vi "Euler Check.vi"(8 "F(X,t)":string[](array[string]), 9 "X":string[](array[string]), 10 "time":string, 11 "X(0)":dbl[](array[numeric]) format="%.2f") -> (0 "system OK":bool, 1 "error text":string[](array[string]), 2 "error":i32[](array[numeric]), 3 "error message":string, 4 "result":dbl[][](array[numeric]), 5 "table":i32[][][](array[numeric]))   [LabVIEW 2014, in "NI_Gmath.lvlib"]
uses:
  NI_Gmath.lvlib
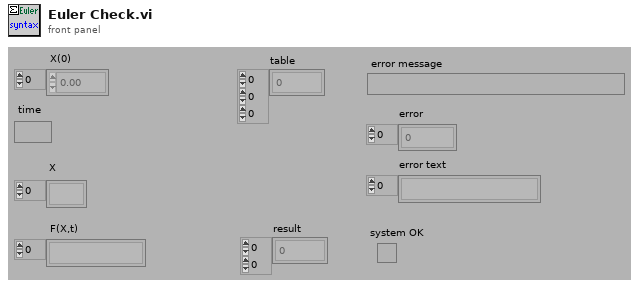
[diagram p1: front panel]
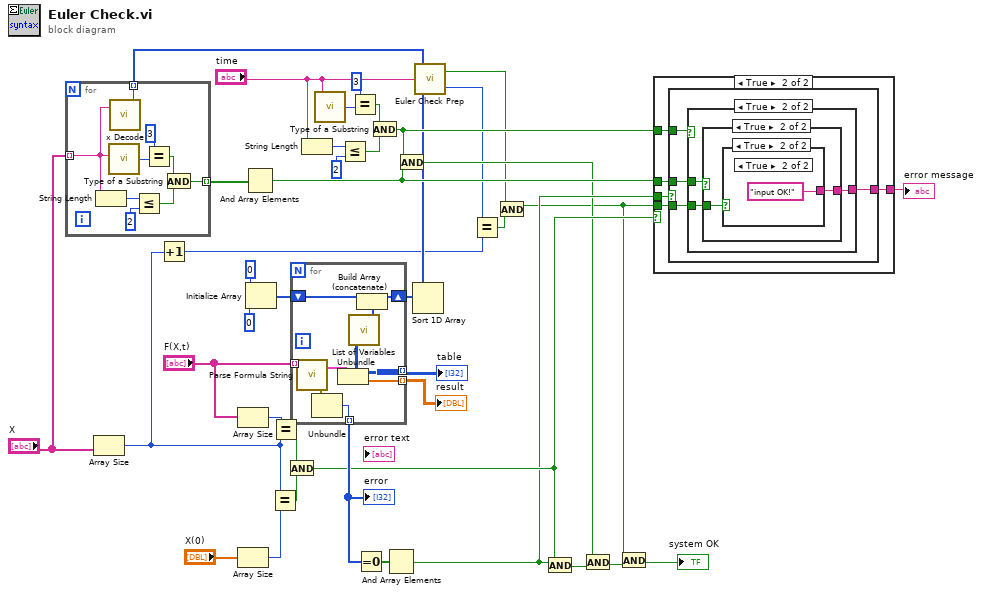
[diagram p0: block diagram]
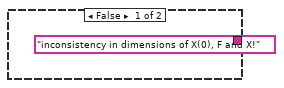
[diagram p2: hidden frame]
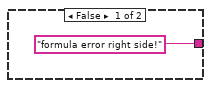
[diagram p3: hidden frame]
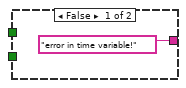
[diagram p4: hidden frame]
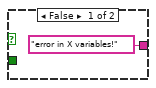
[diagram p5: hidden frame]
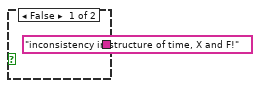
[diagram p6: hidden frame]
diagram:
  n1 = for {
    tunnel: "X" -> [w42] mode=indexing
    tunnel: [w43] -> w21 mode=indexing
    tunnel: [w41] -> w12 mode=indexing
    n2 = String Length(string=w42) -> (length=w44:i32)
    n3 = call "Type of a Substring.VI"("item"=w42) -> ("type"=w46:i32)
    n4 = call "x Decode.vi"("x string"=w42) -> ("number"=w41:i32)  [unwired: 1 in, 1 out]
    n5 = Less Or Equal?(x=w44, y=2) -> (x <= y?=w48:bool)
    n6 = Equal?(x=3, y=w46) -> (x = y?=w49:bool)
    n7 = And(x=w49, y=w48) -> (x .and. y?=w43:bool)
  }
  n8 = Array Size(array="X") -> (size(s)=w11:i32)
  n9 = Increment(x=w11) -> (x+1=w10:i32)
  n10 = Array Size(array="F(X,t)") -> (size(s)=w35:i32)
  n11 = Array Size(array="X(0)") -> (size(s)=w34:i32)
  n12 = And Array Elements(Boolean array=w21) -> (logical AND=w19:bool)
  n13 = Initialize Array(0, 0) -> (w15:i32[])
  n14 = Equal?(x=w11, y=w34) -> (x = y?=w33:bool)
  n15 = Equal?(x=w35, y=w11) -> (x = y?=w32:bool)
  n16 = And(x=w32, y=w33) -> (x .and. y?=w31:bool)
  n17 = for {
    tunnel: [w53] -> w39 mode=indexing
    tunnel: [w51] -> w38 mode=indexing
    tunnel: [w50] -> w37 mode=indexing
    tunnel: "F(X,t)" -> [w58] mode=indexing
    shift-right: [w56] -> w14
    shift-left: w15 -> [w57]
    n18 = call "Parse Formula String.vi"("formula"=w58) -> ("error out"=w54:errorcluster, "Parsed Formula"=w52:cluster{"Table":i32[][], "Y Values":dbl[]})  [unwired: 1 in]
    n19 = Unbundle(w54) -> ("code"=w53:i32)  [unwired: 2 out]
    n20 = Unbundle(w52) -> ("Table"=w51:i32[][], "Y Values"=w50:dbl[])
    n21 = call "List of Variables.vi"("Table"=w51) -> ("List of variables"=w55:i32[])
    n22 = Build Array (concatenate)(w57, w55) -> (w56:i32[])
  }
  "error" <- w39
  "result" <- w37
  "table" <- w38
  n23 = String Length(string="time") -> (length=w28:i32)
  n24 = call "Type of a Substring.VI"("item"="time") -> ("type"=w26:i32)
  n25 = Less Or Equal?(x=w28, y=2) -> (x <= y?=w24:bool)
  n26 = Equal?(x=3, y=w26) -> (x = y?=w23:bool)
  n27 = Equal To 0?(x=w39) -> (x = 0?=w40:bool[])
  n28 = And(x=w23, y=w24) -> (x .and. y?=w20:bool)
  n29 = And Array Elements(Boolean array=w40) -> (logical AND=w29:bool)
  n30 = And(x=w20, y=w19) -> (x .and. y?=w18:bool)
  n31 = Sort 1D Array(array=w14) -> (sorted array=w13:i32[])
  n32 = call "Euler Check Prep.vi"("F(X,t) coded"=w13, "time"="time", "X coded"=w12) -> ("number of X variables"=w9:i32, "variables correct?"=w7:bool)
  n33 = Equal?(x=w9, y=w10) -> (x = y?=w8:bool)
  n34 = And(x=w7, y=w8) -> (x .and. y?=w6:bool)
  n35 = And(x=w31, y=w29) -> (x .and. y?=w22:bool)
  n36 = And(x=w18, y=w22) -> (x .and. y?=w5:bool)
  n37 = And(x=w6, y=w5) -> (x .and. y?=→"system OK":bool)
  n38 = case shown="True" w31 {
    tunnel: ["inconsistency in dimensions of X(0), F and X!" w64] -> w30
    tunnel: w29 -> [_ w63]
    tunnel: w19 -> [_ w62]
    tunnel: w20 -> [_ w61]
    tunnel: w6 -> [_ w60]
    frame False {
    }
    frame True {
      n39 = case shown="True" w63 {
        tunnel: ["formula error right side!" w69] -> w64
        tunnel: w62 -> [_ w68]
        tunnel: w61 -> [_ w67]
        tunnel: w60 -> [_ w66]
        frame False {
        }
        frame True {
          n40 = case shown="True" w67 {
            tunnel: ["error in time variable!" w73] -> w69
            tunnel: w68 -> [_ w72]
            tunnel: w66 -> [_ w71]
            frame False {
            }
            frame True {
              n41 = case shown="True" w72 {
                tunnel: ["error in X variables!" w76] -> w73
                tunnel: w71 -> [_ w75]
                frame False {
                }
                frame True {
                  n42 = case shown="True" w75 {
                    tunnel: ["inconsistency in structure of time, X and F!" "input OK!"] -> w76
                    frame False {
                    }
                    frame True {
                    }
                  }
                }
              }
            }
          }
        }
      }
    }
  }
  "error message" <- w30
